vi "Main.vi"(0 "Credentials":T1) -> (7 "Assets":string[][](table), 8 "Asset Statistics":T2)   [LabVIEW 2020]
doc: "Example usage of HTTP API to communicate with SystemLink Server. This example doest not use LabVIEW-based SystemLink API. Data are taken directly from the SystemLink Server through SystemLink HTTP sAPI."
uses:
  <vilib>/httpClient/LabVIEWHTTPClient.lvlib
panel:
  in  "error in (no error)":errorcluster
  out "error out":errorcluster
  in  "Tab Control":enum32{"Credentials", "Statistics"}(tab)
  # "Instructions:\n1. Insert SystemLink Server IP adress in plain form ex. 127.0.0.1                 2. Insert SystemLink user credentials                                                     3. Run VI                                                                                                     4. Asset data from table will be automatically exported to clipboard"
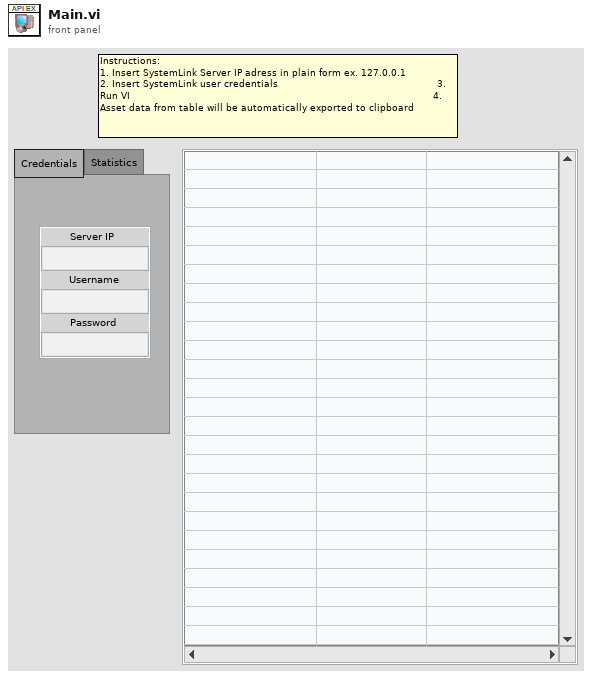
[diagram p1: front panel]
types:
  T1 = cluster{"Server IP":string, "Username":string, "Password":string}
  T2 = cluster{"Systems discovered":i32, "Total Assets":i32, "Active Assets":i32, "Disconnected Assets":i32, "Approaching calibration ":i32, "Past Calibration":i32}
  T3 = typedef "LabVIEWHTTPClient.lvlib/ClientHandle.ctl" = refnum<k1>
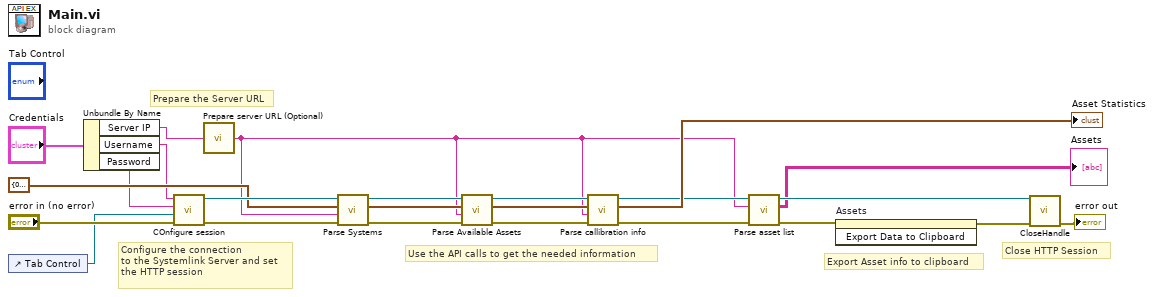
[diagram p0: block diagram]
diagram:
  # "Export Asset info to clipboard"
  # "Close HTTP Session"
  # "Use the API calls to get the needed information"
  # "Prepare the Server URL"
  # "Configure the connection\nto the Systemlink Server and set \nthe HTTP session"
  n1 = control-ref of="Tab Control"() -> (w3:refnum<vi>)
  n2 = Unbundle By Name("Credentials") -> ("Server IP"=w7:string, "Username"=w6:string, "Password"=w5:string)
  n3 = call "COnfigure session.vi"("error in (no error)"="error in (no error)", "Tab control ref"=w3, "password"=w5, "username"=w6) -> ("error out"=w24:errorcluster, "Session out"=w19:T3)  [unwired: 6 in]
  n4 = call "Prepare server URL (Optional).vi"("server url in"=w7) -> ("server url out"=w10:string)
  n5 = call "Parse Systems.vi"("error in (no error)"=w24, "server url in"=w10, "Asset stats in"=T2 {"Systems discovered"=0, "Total Assets"=0, "Active Assets"=0, "Disconnected Assets"=0, "Approaching calibration "=0, "Past Calibration"=8} ("Cluster 2"), "Refnum in"=w19) -> ("error out"=w23:errorcluster, "Asset stats out"=w15:T2, "Refnum out"=w22:T3)  [unwired: 5 in]
  n6 = call "Parse Available Assets.vi"("error in (no error)"=w23, "server url in"=w10, "Statistics in"=w15, "Refnum in"=w22) -> ("error out"=w21:errorcluster, "Statistics out"=w17:T2, "Refnum out"=w20:T3)  [unwired: 5 in]
  n7 = call "Parse callibration info.vi"("Refnum in"=w20, "Statistics in"=w17, "server url in"=w10, "error in (no error)"=w21) -> ("Refnum out"=w13:T3, "Statistics out"=→"Asset Statistics":T2, "error out"=w11:errorcluster)  [unwired: 3 in]
  n8 = call "Parse asset list.vi"("Error in"=w11, "Server URL"=w10, "client handle"=w13) -> ("error out"=w2:errorcluster, "Array"=→"Assets":string[][], "client handle out"=w12:T3)  [unwired: 5 in]
  n9 = invoke on="Assets" class="Tbl (strict)" method="Export Data to Clipboard"(error in=w2) -> (error out=w1:errorcluster)  [unwired: 2 in, 2 out]
  n10 = call <vilib>:"CloseHandle.vi"("client handle"=w12, "error in (no error)"=w1) -> ("error out"=→"error out":errorcluster)  [unwired: 13 in]
